vi "DLS Calc.vi"(9 "Input Bit":T3, 10 "Coeff Data":T2, 11 "DLS ERD Data":T4) -> (3 "Result Q5 Tranformation":dbl)   [LabVIEW 2016, in "TL27.lvlib"]
uses:
  Projects/TL27.lvlib
  Control/DLS ERD Data.ctl
panel:
  out "Result Q5 Tranformation 17":dbl
  out "Result Q5 Tranformation 16":dbl
  out "Result Q5 Tranformation 15":dbl
  out "Result Q5 Tranformation 14":dbl
  out "Result Q5 Tranformation 13":dbl
  out "Result Q5 Tranformation 12":dbl
  out "Result Q5 Tranformation 11":dbl
  out "Result Q5 Tranformation 10":dbl
  out "Result Q5 Tranformation 9":dbl
  out "Result Q5 Tranformation 8":dbl
  out "Result Q5 Tranformation 7":dbl
  out "Result Q5 Tranformation 6":dbl
  out "Result Q5 Tranformation 5":dbl
  out "Result Q5 Tranformation 4":dbl
  out "Result Q5 Tranformation 3":dbl
  out "Result Q5 Tranformation 2":dbl
  out "x*y":dbl
  out "Q":T1
  out "P":T1
  out "O":T1
  out "N":T1
  out "M":T1
  out "L":T1
  out "K":T1
  out "J":T1
  out "I":T1
  out "H":T1
  out "G":T1
  out "F":T1
  out "E":T1
  out "D":T1
  out "C":T1
  out "B":T1
  out "A":T1
  out "Input Bit Q":dbl
  out "Input Bit P":dbl
  out "Input Bit O":dbl
  out "Input Bit N":dbl
  out "Input Bit M":dbl
  out "Input Bit L":dbl
  out "Input Bit K":dbl
  out "Input Bit J":dbl
  out "Input Bit I":dbl
  out "Input Bit H":dbl
  out "Input Bit G":dbl
  out "Input Bit F":dbl
  out "Input Bit E":dbl
  out "Input Bit D":dbl
  out "Input Bit C":dbl
  out "Input Bit B":dbl
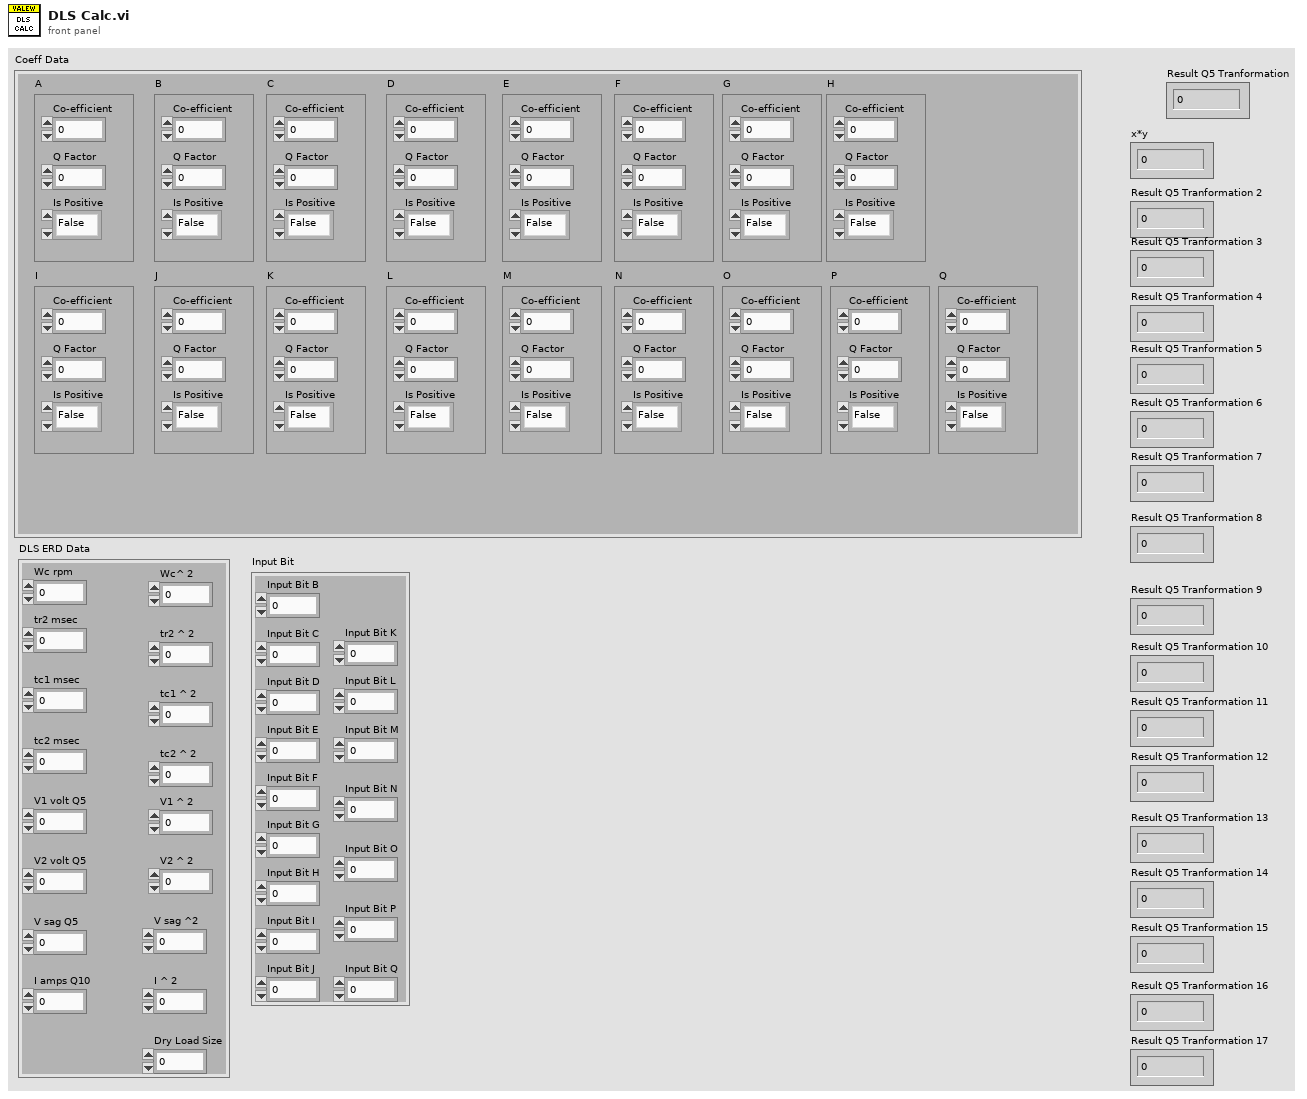
[diagram p1: front panel]
types:
  T1 = cluster{"Co-efficient":dbl, "Q Factor":dbl, "Is Positive":enum16{"False", "True"}}
  T2 = cluster{"A":cluster{"Co-efficient":dbl, "Q Factor":dbl, "Is Positive":enum16{"False", "True"}}, "B":cluster{"Co-efficient":dbl, "Q Factor":dbl, "Is Positive":enum16{"False", "True"}}, "C":cluster{"Co-efficient":dbl, "Q Factor":dbl, "Is Positive":enum16{"False", "True"}}, "D":cluster{"Co-efficient":dbl, "Q Factor":dbl, "Is Positive":enum16{"False", "True"}}, "E":cluster{"Co-efficient":dbl, "Q Factor":dbl, "Is Positive":enum16{"False", "True"}}, "F":cluster{"Co-efficient":dbl, "Q Factor":dbl, "Is Positive":enum16{"False", "True"}}, "G":cluster{"Co-efficient":dbl, "Q Factor":dbl, "Is Positive":enum16{"False", "True"}}, "H":cluster{"Co-efficient":dbl, "Q Factor":dbl, "Is Positive":enum16{"False", "True"}}, "I":cluster{"Co-efficient":dbl, "Q Factor":dbl, "Is Positive":enum16{"False", "True"}}, "J":cluster{"Co-efficient":dbl, "Q Factor":dbl, "Is Positive":enum16{"False", "True"}}, "K":cluster{"Co-efficient":dbl, "Q Factor":dbl, "Is Positive":enum16{"False", "True"}}, "L":cluster{"Co-efficient":dbl, "Q Factor":dbl, "Is Positive":enum16{"False", "True"}}, "M":cluster{"Co-efficient":dbl, "Q Factor":dbl, "Is Positive":enum16{"False", "True"}}, "N":cluster{"Co-efficient":dbl, "Q Factor":dbl, "Is Positive":enum16{"False", "True"}}, "O":cluster{"Co-efficient":dbl, "Q Factor":dbl, "Is Positive":enum16{"False", "True"}}, "P":cluster{"Co-efficient":dbl, "Q Factor":dbl, "Is Positive":enum16{"False", "True"}}, "Q":cluster{"Co-efficient":dbl, "Q Factor":dbl, "Is Positive":enum16{"False", "True"}}}
  T3 = cluster{"Input Bit B":dbl, "Input Bit C":dbl, "Input Bit D":dbl, "Input Bit E":dbl, "Input Bit F":dbl, "Input Bit G":dbl, "Input Bit H":dbl, "Input Bit I":dbl, "Input Bit J":dbl, "Input Bit K":dbl, "Input Bit L":dbl, "Input Bit M":dbl, "Input Bit N":dbl, "Input Bit O":dbl, "Input Bit P":dbl, "Input Bit Q":dbl}
  T4 = typedef "TL27.lvlib/DLS ERD Data.ctl" = cluster{"Wc rpm":dbl, "tr2 msec":dbl, "tc1 msec":dbl, "tc2 msec":dbl, "V1 volt Q5":dbl, "V2 volt Q5":dbl, "I amps Q10":dbl, "Wc^ 2":dbl, "tr2 ^ 2":dbl, "tc1 ^ 2":dbl, "tc2 ^ 2":dbl, "V1 ^ 2":dbl, "V2 ^ 2":dbl, "I ^ 2":dbl, "V sag Q5":dbl, "V sag ^2":dbl, "Dry Load Size":dbl}
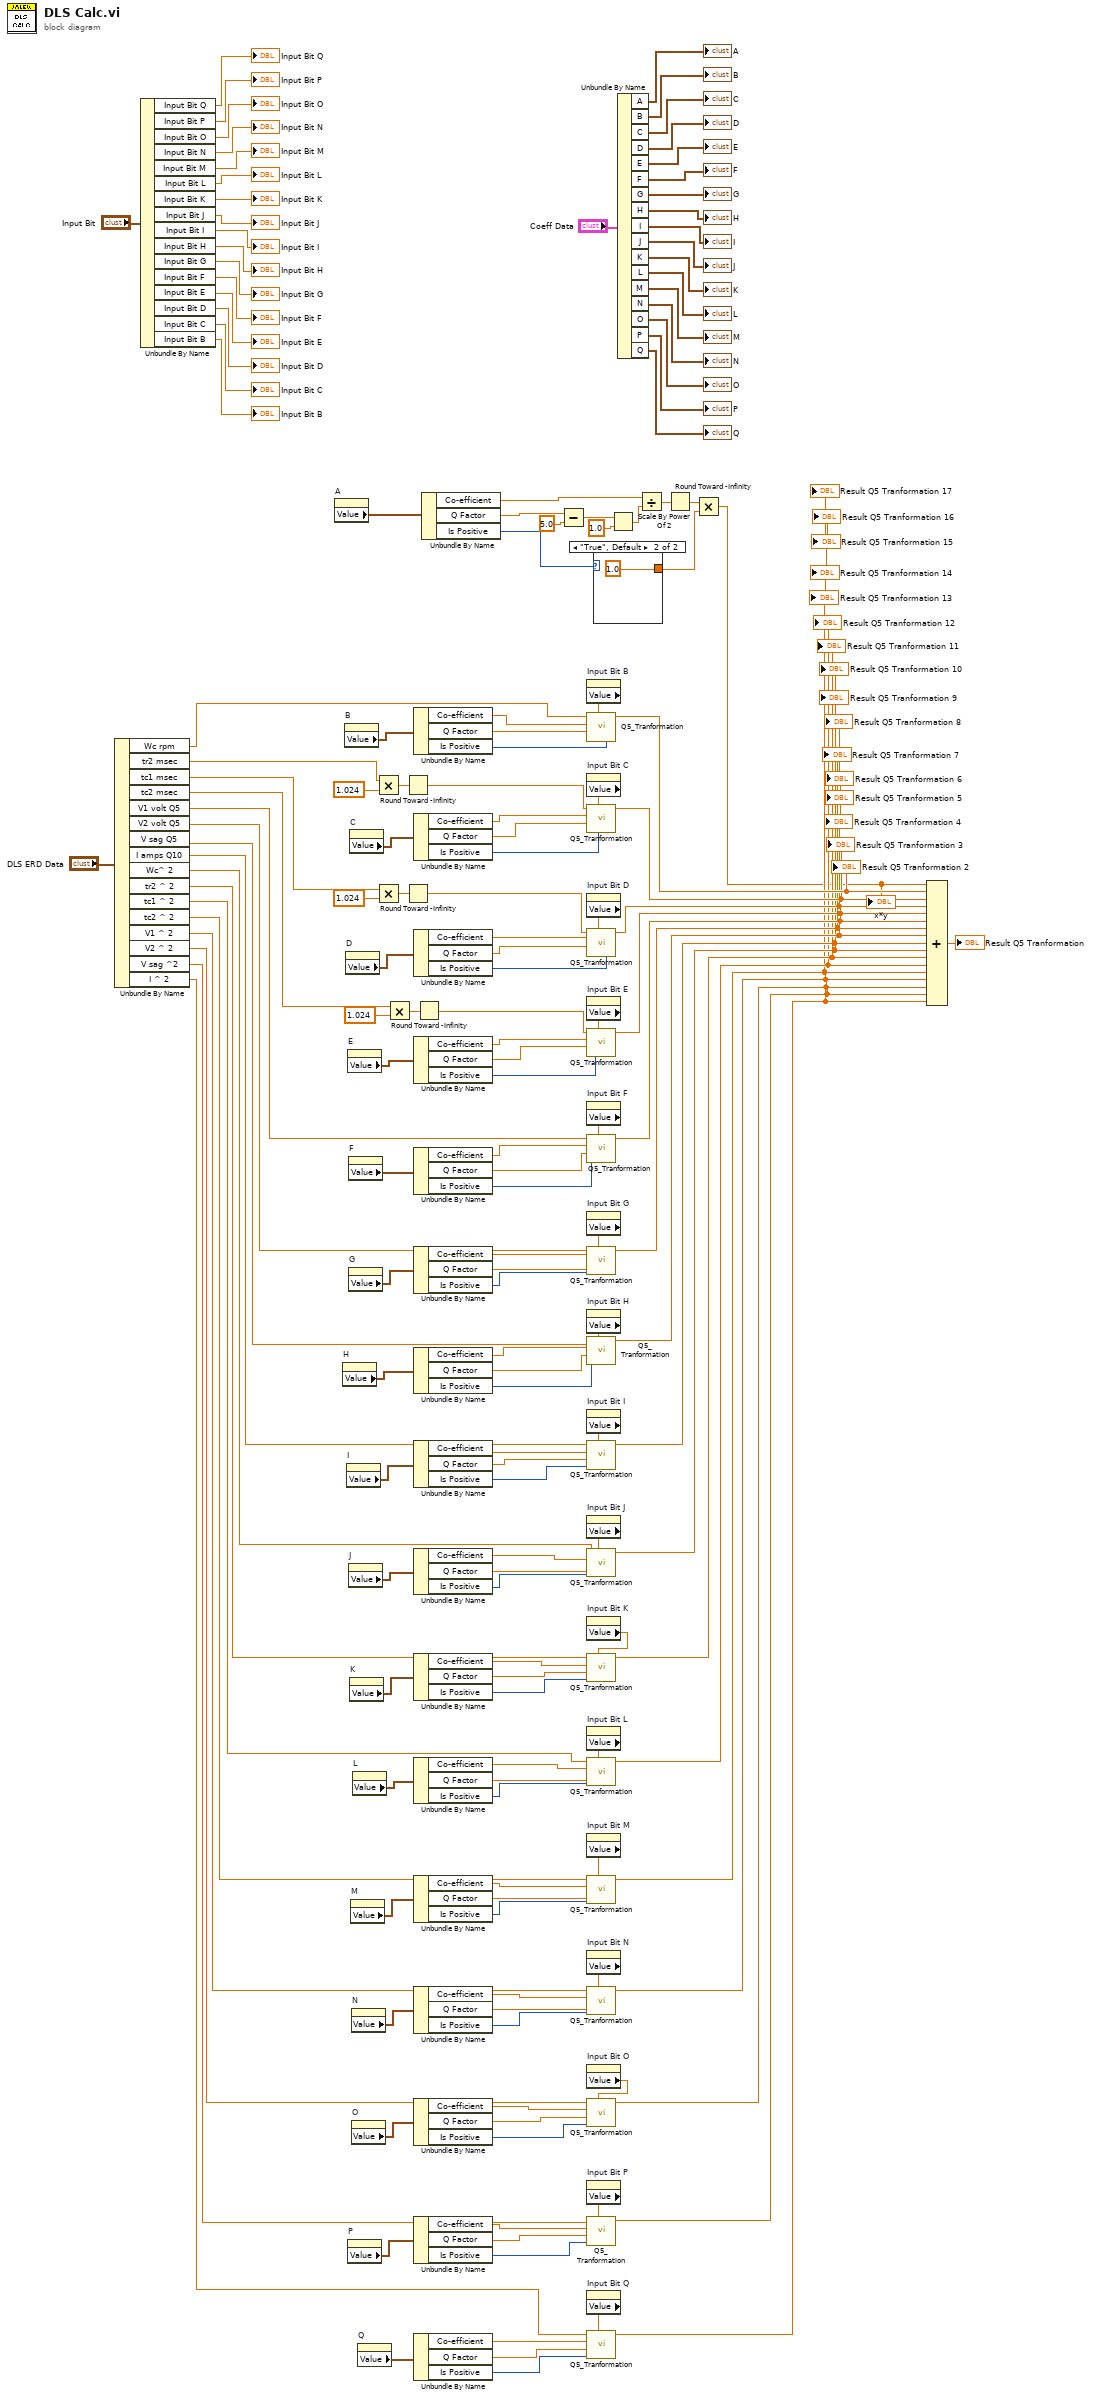
[diagram p0: block diagram]
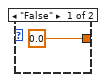
[diagram p2: hidden frame]
diagram:
  n1 = Unbundle By Name("DLS ERD Data") -> ("Wc rpm"=w161:dbl, "tr2 msec"=w12:dbl, "tc1 msec"=w6:dbl, "tc2 msec"=w2:dbl, "V1 volt Q5"=w160:dbl, "V2 volt Q5"=w159:dbl, "V sag Q5"=w158:dbl, "I amps Q10"=w157:dbl, "Wc^ 2"=w156:dbl, "tr2 ^ 2"=w155:dbl, "tc1 ^ 2"=w154:dbl, "tc2 ^ 2"=w153:dbl, "V1 ^ 2"=w152:dbl, "V2 ^ 2"=w151:dbl, "V sag ^2"=w150:dbl, "I ^ 2"=w149:dbl)
  n2 = Unbundle By Name("Input Bit") -> ("Input Bit Q"=→"Input Bit Q":dbl, "Input Bit P"=→"Input Bit P":dbl, "Input Bit O"=→"Input Bit O":dbl, "Input Bit N"=→"Input Bit N":dbl, "Input Bit M"=→"Input Bit M":dbl, "Input Bit L"=→"Input Bit L":dbl, "Input Bit K"=→"Input Bit K":dbl, "Input Bit J"=→"Input Bit J":dbl, "Input Bit I"=→"Input Bit I":dbl, "Input Bit H"=→"Input Bit H":dbl, "Input Bit G"=→"Input Bit G":dbl, "Input Bit F"=→"Input Bit F":dbl, "Input Bit E"=→"Input Bit E":dbl, "Input Bit D"=→"Input Bit D":dbl, "Input Bit C"=→"Input Bit C":dbl, "Input Bit B"=→"Input Bit B":dbl)
  n3 = property on="A" class="Clust (strict)"() -> ("Value"=w47:T1)  [unwired: 2 in, 2 out]
  n4 = property on="H" class="Clust (strict)"() -> ("Value"=w40:T1)  [unwired: 2 in, 2 out]
  n5 = property on="B" class="Clust (strict)"() -> ("Value"=w46:T1)  [unwired: 2 in, 2 out]
  n6 = property on="D" class="Clust (strict)"() -> ("Value"=w44:T1)  [unwired: 2 in, 2 out]
  n7 = property on="I" class="Clust (strict)"() -> ("Value"=w39:T1)  [unwired: 2 in, 2 out]
  n8 = property on="E" class="Clust (strict)"() -> ("Value"=w43:T1)  [unwired: 2 in, 2 out]
  n9 = property on="P" class="Clust (strict)"() -> ("Value"=w32:T1)  [unwired: 2 in, 2 out]
  n10 = property on="F" class="Clust (strict)"() -> ("Value"=w42:T1)  [unwired: 2 in, 2 out]
  n11 = property on="G" class="Clust (strict)"() -> ("Value"=w41:T1)  [unwired: 2 in, 2 out]
  n12 = property on="J" class="Clust (strict)"() -> ("Value"=w38:T1)  [unwired: 2 in, 2 out]
  n13 = property on="C" class="Clust (strict)"() -> ("Value"=w45:T1)  [unwired: 2 in, 2 out]
  n14 = property on="K" class="Clust (strict)"() -> ("Value"=w37:T1)  [unwired: 2 in, 2 out]
  n15 = property on="M" class="Clust (strict)"() -> ("Value"=w35:T1)  [unwired: 2 in, 2 out]
  n16 = property on="N" class="Clust (strict)"() -> ("Value"=w34:T1)  [unwired: 2 in, 2 out]
  n17 = property on="O" class="Clust (strict)"() -> ("Value"=w33:T1)  [unwired: 2 in, 2 out]
  n18 = property on="L" class="Clust (strict)"() -> ("Value"=w36:T1)  [unwired: 2 in, 2 out]
  n19 = property on="Q" class="Clust (strict)"() -> ("Value"=w31:T1)  [unwired: 2 in, 2 out]
  n20 = Multiply(x=w12, y=1.024) -> (x*y=w10:dbl)
  n21 = Multiply(x=w6, y=1.024) -> (x*y=w7:dbl)
  n22 = Multiply(x=w2, y=1.024) -> (x*y=w4:dbl)
  n23 = Round Toward -Infinity(1:w10) -> (0:w9:dbl)
  n24 = Round Toward -Infinity(1:w7) -> (0:w5:dbl)
  n25 = Unbundle By Name(w46) -> ("Co-efficient"=w170:dbl, "Q Factor"=w169:dbl, "Is Positive"=w168:enum16{"False", "True"})
  n26 = Unbundle By Name(w45) -> ("Co-efficient"=w165:dbl, "Q Factor"=w166:dbl, "Is Positive"=w167:enum16{"False", "True"})
  n27 = Unbundle By Name(w44) -> ("Co-efficient"=w144:dbl, "Q Factor"=w143:dbl, "Is Positive"=w148:enum16{"False", "True"})
  n28 = Unbundle By Name(w43) -> ("Co-efficient"=w146:dbl, "Q Factor"=w145:dbl, "Is Positive"=w147:enum16{"False", "True"})
  n29 = Unbundle By Name(w42) -> ("Co-efficient"=w108:dbl, "Q Factor"=w142:dbl, "Is Positive"=w76:enum16{"False", "True"})
  n30 = Unbundle By Name(w41) -> ("Co-efficient"=w141:dbl, "Q Factor"=w140:dbl, "Is Positive"=w139:enum16{"False", "True"})
  n31 = Unbundle By Name(w40) -> ("Co-efficient"=w138:dbl, "Q Factor"=w137:dbl, "Is Positive"=w136:enum16{"False", "True"})
  n32 = Unbundle By Name(w39) -> ("Co-efficient"=w135:dbl, "Q Factor"=w134:dbl, "Is Positive"=w133:enum16{"False", "True"})
  n33 = Unbundle By Name(w38) -> ("Co-efficient"=w132:dbl, "Q Factor"=w131:dbl, "Is Positive"=w130:enum16{"False", "True"})
  n34 = Unbundle By Name(w37) -> ("Co-efficient"=w129:dbl, "Q Factor"=w128:dbl, "Is Positive"=w127:enum16{"False", "True"})
  n35 = Unbundle By Name(w36) -> ("Co-efficient"=w126:dbl, "Q Factor"=w125:dbl, "Is Positive"=w124:enum16{"False", "True"})
  n36 = Unbundle By Name(w35) -> ("Co-efficient"=w123:dbl, "Q Factor"=w122:dbl, "Is Positive"=w121:enum16{"False", "True"})
  n37 = Unbundle By Name(w34) -> ("Co-efficient"=w120:dbl, "Q Factor"=w119:dbl, "Is Positive"=w118:enum16{"False", "True"})
  n38 = Unbundle By Name(w33) -> ("Co-efficient"=w117:dbl, "Q Factor"=w116:dbl, "Is Positive"=w115:enum16{"False", "True"})
  n39 = Unbundle By Name(w32) -> ("Co-efficient"=w114:dbl, "Q Factor"=w113:dbl, "Is Positive"=w112:enum16{"False", "True"})
  n40 = Unbundle By Name(w31) -> ("Co-efficient"=w111:dbl, "Q Factor"=w110:dbl, "Is Positive"=w109:enum16{"False", "True"})
  n41 = Round Toward -Infinity(1:w4) -> (0:w1:dbl)
  n42 = Unbundle By Name(w47) -> ("Co-efficient"=w54:dbl, "Q Factor"=w57:dbl, "Is Positive"=w50:enum16{"False", "True"})
  n43 = Subtract(x=w57, y=5.0) -> (x-y=w55:dbl)
  n44 = property on="Input Bit B" class="DigNum (strict)"() -> ("Value"=w107:dbl)  [unwired: 2 in, 2 out]
  n45 = call "Q5_Tranformation.vi"("Input Bit"=w107, "Is Positive"=w168, "Q Factor"=w169, "Coefficient"=w170, "DLS ERD Data"=w161) -> ("Result Q5 Tranformation"=w75:dbl)  [unwired: 6 in]
  "Result Q5 Tranformation 2" <- w75
  n46 = property on="Input Bit C" class="DigNum (strict)"() -> ("Value"=w91:dbl)  [unwired: 2 in, 2 out]
  n47 = call "Q5_Tranformation.vi"("Input Bit"=w91, "Is Positive"=w167, "Q Factor"=w166, "Coefficient"=w165, "DLS ERD Data"=w9) -> ("Result Q5 Tranformation"=w74:dbl)  [unwired: 6 in]
  "Result Q5 Tranformation 3" <- w74
  n48 = property on="Input Bit D" class="DigNum (strict)"() -> ("Value"=w90:dbl)  [unwired: 2 in, 2 out]
  n49 = call "Q5_Tranformation.vi"("Input Bit"=w90, "Is Positive"=w148, "Q Factor"=w143, "Coefficient"=w144, "DLS ERD Data"=w5) -> ("Result Q5 Tranformation"=w73:dbl)  [unwired: 6 in]
  "Result Q5 Tranformation 4" <- w73
  n50 = property on="Input Bit E" class="DigNum (strict)"() -> ("Value"=w89:dbl)  [unwired: 2 in, 2 out]
  n51 = call "Q5_Tranformation.vi"("Input Bit"=w89, "Is Positive"=w147, "Q Factor"=w145, "Coefficient"=w146, "DLS ERD Data"=w1) -> ("Result Q5 Tranformation"=w72:dbl)  [unwired: 6 in]
  "Result Q5 Tranformation 5" <- w72
  n52 = property on="Input Bit F" class="DigNum (strict)"() -> ("Value"=w88:dbl)  [unwired: 2 in, 2 out]
  n53 = call "Q5_Tranformation.vi"("Input Bit"=w88, "Is Positive"=w76, "Q Factor"=w142, "Coefficient"=w108, "DLS ERD Data"=w160) -> ("Result Q5 Tranformation"=w71:dbl)  [unwired: 6 in]
  "Result Q5 Tranformation 6" <- w71
  n54 = property on="Input Bit G" class="DigNum (strict)"() -> ("Value"=w87:dbl)  [unwired: 2 in, 2 out]
  n55 = call "Q5_Tranformation.vi"("Input Bit"=w87, "Is Positive"=w139, "Q Factor"=w140, "Coefficient"=w141, "DLS ERD Data"=w159) -> ("Result Q5 Tranformation"=w70:dbl)  [unwired: 6 in]
  "Result Q5 Tranformation 7" <- w70
  n56 = property on="Input Bit H" class="DigNum (strict)"() -> ("Value"=w86:dbl)  [unwired: 2 in, 2 out]
  n57 = call "Q5_Tranformation.vi"("Input Bit"=w86, "Is Positive"=w136, "Q Factor"=w137, "Coefficient"=w138, "DLS ERD Data"=w158) -> ("Result Q5 Tranformation"=w69:dbl)  [unwired: 6 in]
  "Result Q5 Tranformation 8" <- w69
  n58 = property on="Input Bit I" class="DigNum (strict)"() -> ("Value"=w85:dbl)  [unwired: 2 in, 2 out]
  n59 = call "Q5_Tranformation.vi"("Input Bit"=w85, "Is Positive"=w133, "Q Factor"=w134, "Coefficient"=w135, "DLS ERD Data"=w157) -> ("Result Q5 Tranformation"=w68:dbl)  [unwired: 6 in]
  "Result Q5 Tranformation 9" <- w68
  n60 = property on="Input Bit J" class="DigNum (strict)"() -> ("Value"=w84:dbl)  [unwired: 2 in, 2 out]
  n61 = call "Q5_Tranformation.vi"("Input Bit"=w84, "Is Positive"=w130, "Q Factor"=w131, "Coefficient"=w132, "DLS ERD Data"=w156) -> ("Result Q5 Tranformation"=w67:dbl)  [unwired: 6 in]
  "Result Q5 Tranformation 10" <- w67
  n62 = property on="Input Bit K" class="DigNum (strict)"() -> ("Value"=w83:dbl)  [unwired: 2 in, 2 out]
  n63 = call "Q5_Tranformation.vi"("Input Bit"=w83, "Is Positive"=w127, "Q Factor"=w128, "Coefficient"=w129, "DLS ERD Data"=w155) -> ("Result Q5 Tranformation"=w66:dbl)  [unwired: 6 in]
  "Result Q5 Tranformation 11" <- w66
  n64 = property on="Input Bit L" class="DigNum (strict)"() -> ("Value"=w82:dbl)  [unwired: 2 in, 2 out]
  n65 = call "Q5_Tranformation.vi"("Input Bit"=w82, "Is Positive"=w124, "Q Factor"=w125, "Coefficient"=w126, "DLS ERD Data"=w154) -> ("Result Q5 Tranformation"=w65:dbl)  [unwired: 6 in]
  "Result Q5 Tranformation 12" <- w65
  n66 = property on="Input Bit M" class="DigNum (strict)"() -> ("Value"=w81:dbl)  [unwired: 2 in, 2 out]
  n67 = call "Q5_Tranformation.vi"("Input Bit"=w81, "Is Positive"=w121, "Q Factor"=w122, "Coefficient"=w123, "DLS ERD Data"=w153) -> ("Result Q5 Tranformation"=w64:dbl)  [unwired: 6 in]
  "Result Q5 Tranformation 13" <- w64
  n68 = property on="Input Bit N" class="DigNum (strict)"() -> ("Value"=w80:dbl)  [unwired: 2 in, 2 out]
  n69 = call "Q5_Tranformation.vi"("Input Bit"=w80, "Is Positive"=w118, "Q Factor"=w119, "Coefficient"=w120, "DLS ERD Data"=w152) -> ("Result Q5 Tranformation"=w63:dbl)  [unwired: 6 in]
  "Result Q5 Tranformation 14" <- w63
  n70 = property on="Input Bit O" class="DigNum (strict)"() -> ("Value"=w79:dbl)  [unwired: 2 in, 2 out]
  n71 = call "Q5_Tranformation.vi"("Input Bit"=w79, "Is Positive"=w115, "Q Factor"=w116, "Coefficient"=w117, "DLS ERD Data"=w151) -> ("Result Q5 Tranformation"=w62:dbl)  [unwired: 6 in]
  "Result Q5 Tranformation 15" <- w62
  n72 = property on="Input Bit P" class="DigNum (strict)"() -> ("Value"=w78:dbl)  [unwired: 2 in, 2 out]
  n73 = call "Q5_Tranformation.vi"("Input Bit"=w78, "Is Positive"=w112, "Q Factor"=w113, "Coefficient"=w114, "DLS ERD Data"=w150) -> ("Result Q5 Tranformation"=w61:dbl)  [unwired: 6 in]
  "Result Q5 Tranformation 16" <- w61
  n74 = property on="Input Bit Q" class="DigNum (strict)"() -> ("Value"=w77:dbl)  [unwired: 2 in, 2 out]
  n75 = call "Q5_Tranformation.vi"("Input Bit"=w77, "Is Positive"=w109, "Q Factor"=w110, "Coefficient"=w111, "DLS ERD Data"=w149) -> ("Result Q5 Tranformation"=w60:dbl)  [unwired: 6 in]
  "Result Q5 Tranformation 17" <- w60
  n76 = case shown="\"True\", Default" w50 {
    tunnel: [0.0 1.0] -> w49
    frame "False" {
    }
    frame "True", Default {
    }
  }
  n77 = Scale By Power Of 2(n=w55, x=1.0) -> (x*2^n=w53:dbl)
  n78 = Unbundle By Name("Coeff Data") -> ("A"=→"A":T1, "B"=→"B":T1, "C"=→"C":T1, "D"=→"D":T1, "E"=→"E":T1, "F"=→"F":T1, "G"=→"G":T1, "H"=→"H":T1, "I"=→"I":T1, "J"=→"J":T1, "K"=→"K":T1, "L"=→"L":T1, "M"=→"M":T1, "N"=→"N":T1, "O"=→"O":T1, "P"=→"P":T1, "Q"=→"Q":T1)
  n79 = Divide(x=w54, y=w53) -> (x/y=w52:dbl)
  n80 = Round Toward -Infinity(1:w52) -> (0:w51:dbl)
  n81 = Multiply(x=w51, y=w49) -> (x*y=w48:dbl)
  "x*y" <- w48
  n82 = Compound Arithmetic op=ADD(w48, w75, w74, w73, w72, w71, w70, w69, w68, w67, w66, w65, w64, w63, w62, w61, w60) -> (→"Result Q5 Tranformation":dbl)
